vi "Initialize.vi"(8 "error in (no error)":errorcluster, 11 "S4ACS_GUI in":refnum<class "GuiderSetup.lvclass">) -> (0 "error out":errorcluster, 3 "S4ACS_GUI out":refnum<class "GuiderSetup.lvclass">)   [LabVIEW 2018, in "GuiderSetup.lvclass"]
uses:
  GuiderSetup.lvclass
  C:/Users/observer/Desktop/Sparc4GUI/Versao ZeroMQ/SPARC4_GUI/S4GUI/S4GUI.lvclass
  S4GUI/S4GUI.lvclass/S4GUI.ctl
  GuiderSetup.lvclass/GuiderSetup.ctl
  Instrument/Instrument.lvclass
  AG/AG.lvclass
  S4GUI/S4GUI.lvclass
panel:
  in  "Guider Status":cluster{"AG status":bool, "rotator":dbl}
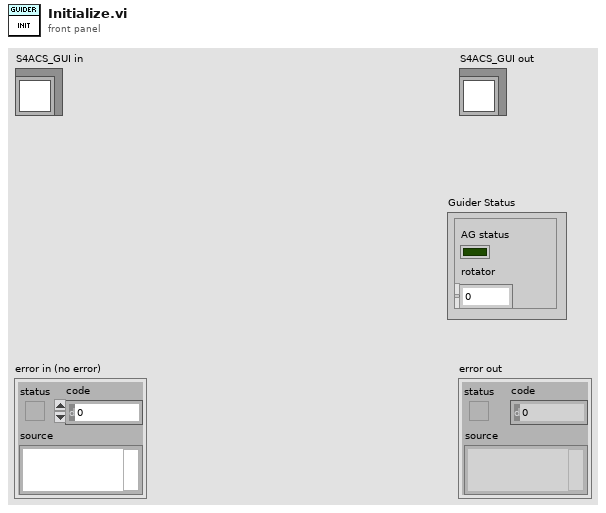
[diagram p1: front panel]
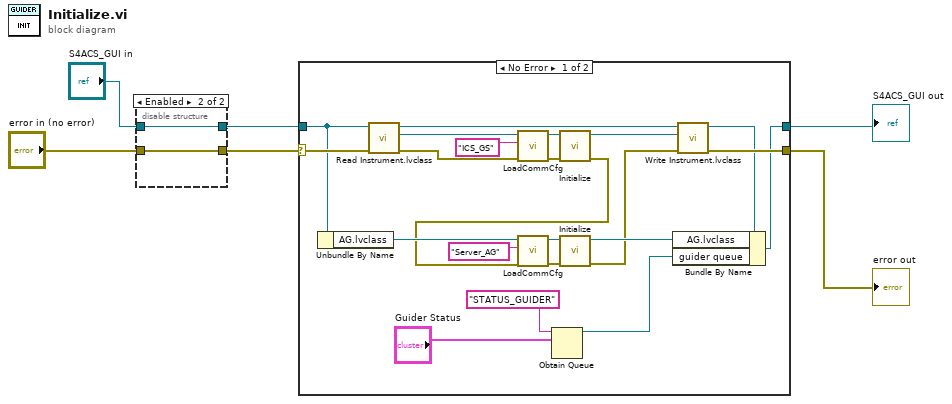
[diagram p0: block diagram]
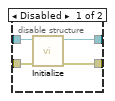
[diagram p2: hidden frame]
diagram:
  n1 = disable-structure shown="Enabled" {
    disable-tunnel: "error in (no error)" -> [w10 w11]
    disable-tunnel: "S4ACS_GUI in" -> [w9 w12]
    disable-tunnel: [w8 w12] -> w4
    disable-tunnel: [w7 w11] -> w3
    frame Disabled {
      n2 = call-parent "Initialize.vi"("error in (no error)"=w10, "S4ACS_GUI in"=w9) -> ("error out"=w7:errorcluster, "S4ACS_GUI out"=w8:refnum<class "GuiderSetup.lvclass">)  [unwired: 8 in]
    }
    frame Enabled {
    }
  }
  n3 = case shown="No Error" w3 {
    selector: w3 -> [w34 w35]
    tunnel: w4 -> [w30 w36]
    tunnel: [w31 w35] -> w1
    tunnel: [w27 w36] -> w2
    frame No Error {
      n4 = Unbundle By Name(w30) -> ("AG.lvclass"=w18:refnum<class "AG.lvclass">)
      n5 = call "Read Instrument.lvclass.vi"("error in (no error)"=w34, "S4ACS_GUI in"=w30) -> ("error out"=w21:errorcluster, "Instrument.lvclass"=w22:refnum<class "Instrument.lvclass">, "S4ACS_GUI out"=w32:refnum<class "GuiderSetup.lvclass">)  [unwired: 7 in]
      n6 = call-dynamic "LoadCommCfg.vi"("error in (no error)"=w21, "section (server name)"="ICS_GS", "Server in"=w22) -> ("error out"=w20:errorcluster, "Server out"=w19:refnum<class "Instrument.lvclass">)  [unwired: 7 in]
      n7 = Obtain Queue(name (unnamed)="STATUS_GUIDER", element data type="Guider Status") -> (queue out=w23:refnum<queue>)  [unwired: 3 in, 2 out]
      n8 = call-dynamic "Initialize.vi"("error in (no error)"=w20, "Instrument in"=w19) -> ("error out"=w15:errorcluster, "Instrument out"=w33:refnum<class "Instrument.lvclass">)  [unwired: 8 in]
      n9 = call-dynamic "LoadCommCfg.vi"("error in (no error)"=w15, "section (server name)"="Server_AG", "Server in"=w18) -> ("error out"=w16:errorcluster, "Server out"=w17:refnum<class "AG.lvclass">)  [unwired: 7 in]
      n10 = call-dynamic "Initialize.vi"("error in (no error)"=w16, "AG in"=w17) -> ("error out"=w26:errorcluster, "AG out"=w28:refnum<class "AG.lvclass">)  [unwired: 8 in]
      n11 = call "Write Instrument.lvclass.vi"("error in (no error)"=w26, "Instrument.lvclass"=w33, "S4ACS_GUI in"=w32) -> ("error out"=w31:errorcluster, "S4ACS_GUI out"=w29:refnum<class "GuiderSetup.lvclass">)  [unwired: 7 in]
      n12 = Bundle By Name(cluster=w29, "AG.lvclass"=w28, "guider queue"=w23) -> (w27:refnum<class "GuiderSetup.lvclass">)
    }
    frame Error {
    }
  }
  "error out" <- w1
  "S4ACS_GUI out" <- w2
